vi "Set Pixel (RGBA).vi"(4 "Error":string, 5 "Pixel":T1, 6 "Y":i32, 7 "X":i32, 8 "Image":T2={"Image ID"=0, "Channel ID"=-1}) -> (0 "Error":string, 3 "Image":T2={"Image ID"=0, "Channel ID"=-1})   [LabVIEW 2011, in "labvvis.lvlib"]
doc: "Changes the value of the pixel in Image, at the position (X, Y) to the RGBA pixel specified by Red, Green, Blue and Alpha. This version is only applicable to RGBA images."
uses:
  <userlib>/labvvis/labvvis.lvlib
  <userlib>/labvvis/VVIS Image.ctl
  <userlib>/labvvis/RGBA Pixel.ctl
  labvvis.framework
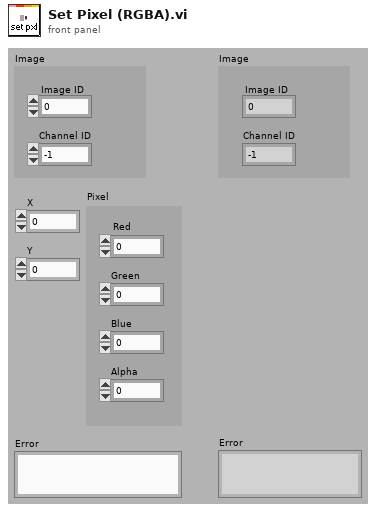
[diagram p1: front panel]
types:
  T1 = typedef "labvvis.lvlib/RGBA Pixel.ctl" = cluster{"Red ":u8, "Green":u8, "Blue":u8, "Alpha":u8}
  T2 = typedef "labvvis.lvlib/VVIS Image.ctl" = cluster{"Image ID":i16, "Channel ID":i16}
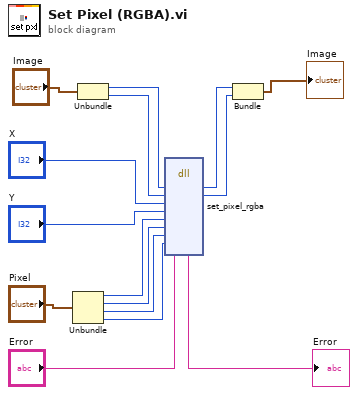
[diagram p0: block diagram]
diagram:
  n1 = Unbundle("Pixel") -> ("Red"=w8:u8, "Green"=w7:u8, "Blue"=w6:u8, "Alpha"=w5:u8)
  n2 = Unbundle("Image") -> ("Image ID"=w12:i16, "Channel ID"=w11:i16)
  n3 = dll-call lib="labvvis.framework" fn="set_pixel_rgba"("out"=w12, "cid"=w11, "x"="X", "y"="Y", "r"=w8, "g"=w7, "b"=w6, "a"=w5, "error"="Error") -> ("out"=w14:i16, "cid"=w2:i16, "error"=→"Error":string)  [unwired: 10 in, 2 out]
  n4 = Bundle("out"=w14, "cid"=w2) -> (→"Image":cluster{"out":i16, "cid":i16})  [unwired: 1 in]
